vi "Time Since Calibration.vi"(8 "Error In":errorcluster) -> (0 "Error Out":errorcluster, 1 "Time Since Last Calibration (Weeks)":dbl, 2 "Time Since Last Calibration (Days)":dbl, 3 "Time Since Last Calibration (Hours)":dbl)   [LabVIEW 2019, in "SubVIs.lvlib"]
uses:
  SubVIs.lvlib
panel:
  out "Time Since Last Calibration (Months)":dbl
  out "Time Since Last Calibration (Miutes)":dbl
  out "Time Since Last Calibration (Seconds)":dbl
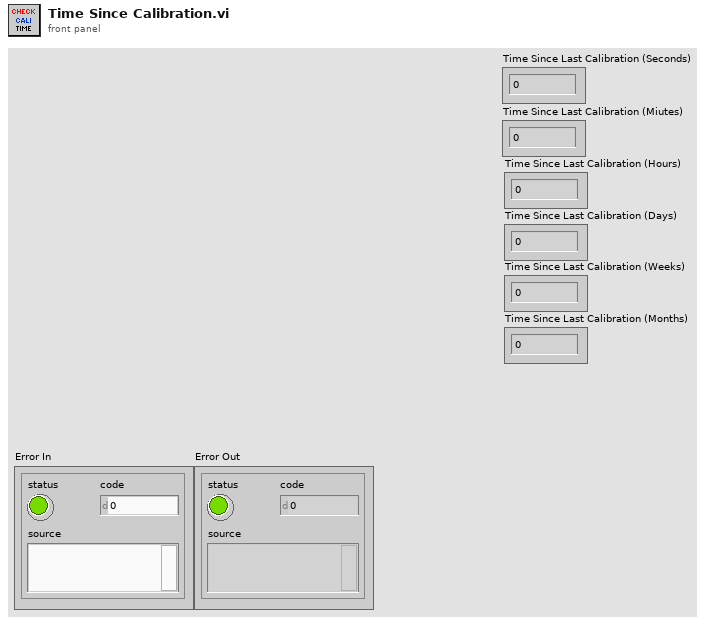
[diagram p1: front panel]
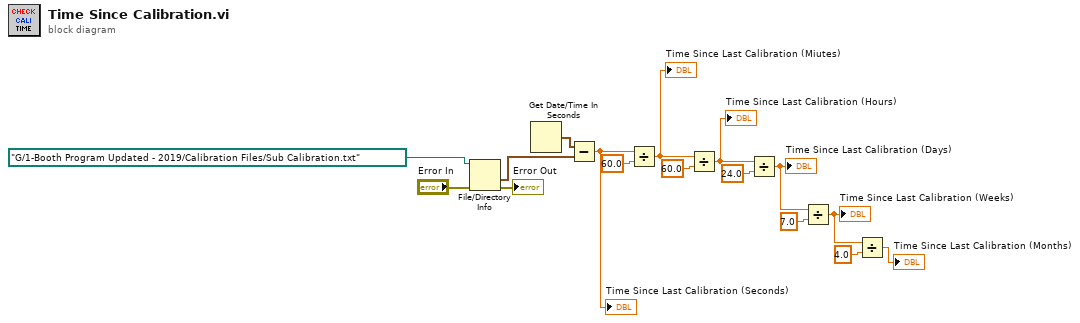
[diagram p0: block diagram]
diagram:
  n1 = File/Directory Info(path=path "G:/1-Booth Program Updated - 2019/Calibration Files/Sub Calibration.txt" ("file path (use dialog)"), error in="Error In") -> (last mod=w13:timestamp, error out=→"Error Out":errorcluster)  [unwired: 5 out]
  n2 = Get Date/Time In Seconds() -> (seconds since 1Jan1904=w14:timestamp)
  n3 = Subtract(x=w14, y=w13) -> (x-y=w11:dbl)
  "Time Since Last Calibration (Seconds)" <- w11
  n4 = Divide(x=w11, y=60.0) -> (x/y=w9:dbl)
  "Time Since Last Calibration (Miutes)" <- w9
  n5 = Divide(x=w9, y=60.0) -> (x/y=w7:dbl)
  "Time Since Last Calibration (Hours)" <- w7
  n6 = Divide(x=w7, y=24.0) -> (x/y=w5:dbl)
  "Time Since Last Calibration (Days)" <- w5
  n7 = Divide(x=w5, y=7.0) -> (x/y=w3:dbl)
  "Time Since Last Calibration (Weeks)" <- w3
  n8 = Divide(x=w3, y=4.0) -> (x/y=→"Time Since Last Calibration (Months)":dbl)
